vi "Update Head Worker Symbol.vi"(6 "Connected?":bool, 8 "error in (no error)":errorcluster, 9 "WID":string, 10 "DC_UID":T1, 11 "Tree Ref":refnum<vi>) -> (0 "error out":errorcluster)   [LabVIEW 2017, in "Application Manager.lvclass"]
uses:
  Application Manager.lvclass
  Common VIs/DC_UID.ctl
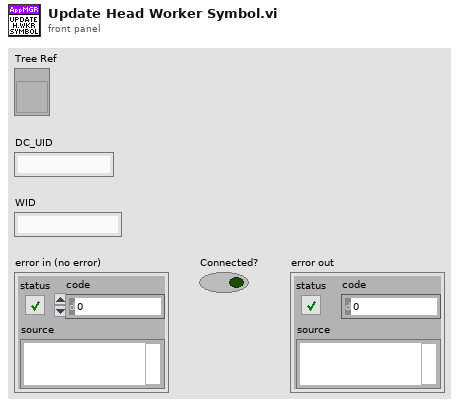
[diagram p1: front panel]
types:
  T1 = typedef "DC_UID.ctl" = string
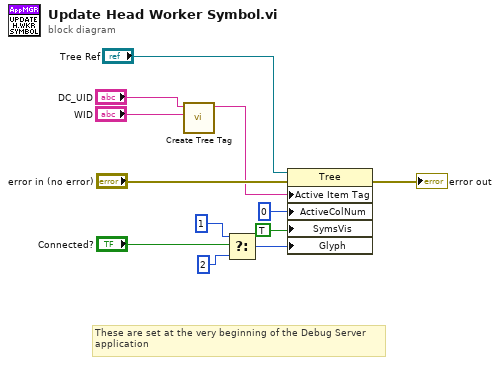
[diagram p0: block diagram]
diagram:
  # "These are set at the very beginning of the Debug Server\napplication"
  n1 = call "Create Tree Tag.vi"("WID"="WID", "DC_UID"="DC_UID") -> ("Tree Tag"=w2:string)  [unwired: 9 in]
  n2 = Select(t=1 ("Active Item:Symbol Index"), s="Connected?", f=2 ("Active Item:Symbol Index")) -> (s? t:f=w10:i32)
  n3 = property class="Tree"(reference="Tree Ref", error in="error in (no error)", "Active Item Tag"=w2, "ActiveColNum"=0 ("Active Cell:Active Column Number"), "SymsVis"=TRUE ("Visible Items:Symbols Visible"), "Glyph"=w10) -> (error out=→"error out":errorcluster)  [unwired: 1 out]
